vi "Joystick Sensitivity.vi"(9 "Throtle (0 to +1)":dbl min=0.0 max=1.0 step=0.1 format="%#_5g", 11 "Joystick Output (-1 to +1)":dbl min=-1.0 max=1.0 step=0.1 format="%#_5g") -> (3 "Sensitivity Adjusted Output (-1 to +1)":dbl min=-1.0 max=1.0 format="%#_5g")   [LabVIEW 2017]
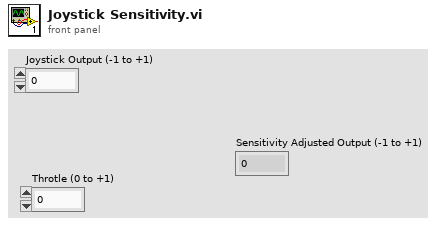
[diagram p1: front panel]
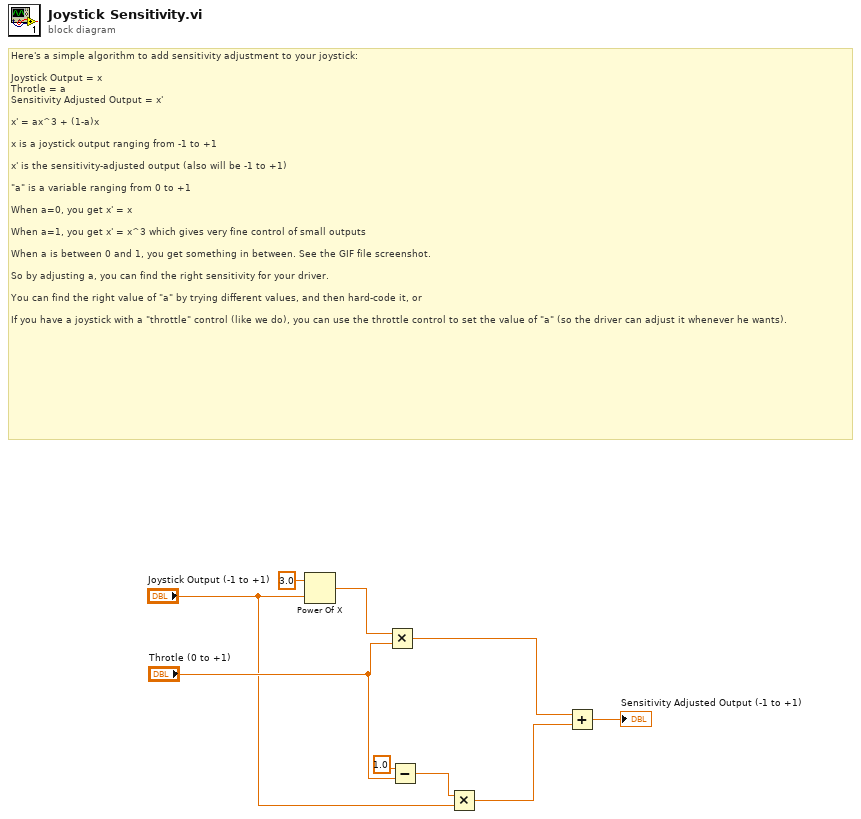
[diagram p0: block diagram]
diagram:
  # "Here's a simple algorithm to add sensitivity adjustment to your joystick:\n\nJoystick Output = x\nThrotle = a\nSensitivity Adjusted Output = x'\n\nx' = ax^3 + (1-a)x\n\nx is a joystick output ranging from -1 to +1\n\nx' is the sensitivity-adjusted output (also will be -1 to +1)\n\n\"a\" is a variable ranging from 0 to +1\n\nWhen a=0, you get x' = x\n\nWhen a=1, you get x' = x^3 which gives very fine control of small outputs\n\nWhen a is between 0 and 1, you get something in between. See the GIF file screenshot.\n\nSo by adjusting a, you can find the right sensitivity for your driver.\n\nYou can find the right value of \"a\" by trying different values, and then hard-code it, or\n\nIf you have a joystick with a \"throttle\" control (like we do), you can use the throttle control to set the value of \"a\" (so the driver can adjust it whenever he wants)."
  n1 = Power Of X(1:"Joystick Output (-1 to +1)", 2:3.0 ("y")) -> (0:w8:dbl)
  n2 = Multiply(x=w8, y="Throtle (0 to +1)") -> (x*y=w7:dbl)
  n3 = Subtract(x=1.0, y="Throtle (0 to +1)") -> (x-y=w4:dbl)
  n4 = Multiply(x=w4, y="Joystick Output (-1 to +1)") -> (x*y=w2:dbl)
  n5 = Add(x=w7, y=w2) -> (x+y=→"Sensitivity Adjusted Output (-1 to +1)":dbl)
